vi "HMI_GetPaths.vi"(11 "Main Root Path":path) -> (1 "Default Paths":path[](array[path])=[path "C:/AllenProjects/PWC-OLS/$ReportFiles", path "C:/AllenProjects/PWC-OLS/$ConfigFiles"], 2 "Root Path":path=path "C:/AllenProjects/PWC-OLS", 3 "vi path":path)   [LabVIEW 2024]
doc: "Use to create relative paths to make the program portable.I\n\niNPUTS\nRelative Path is the name of the folder where to begin the file open dialog.\nRoot Name is the String name of the Root folder of this program.\n\nOUTPUS\nFile Path Path to the Opened File\nRoot Path Path to the root Folder\nFile Name String name less Path and extension."
panel:
  in  "Default Relative Paths":path[](array[path])=[path "$ReportFiles", path "$ConfigFiles"]
  in  "Reg Key Srting":string[](array[string])=["Report Files Path", "Config Files Path"]
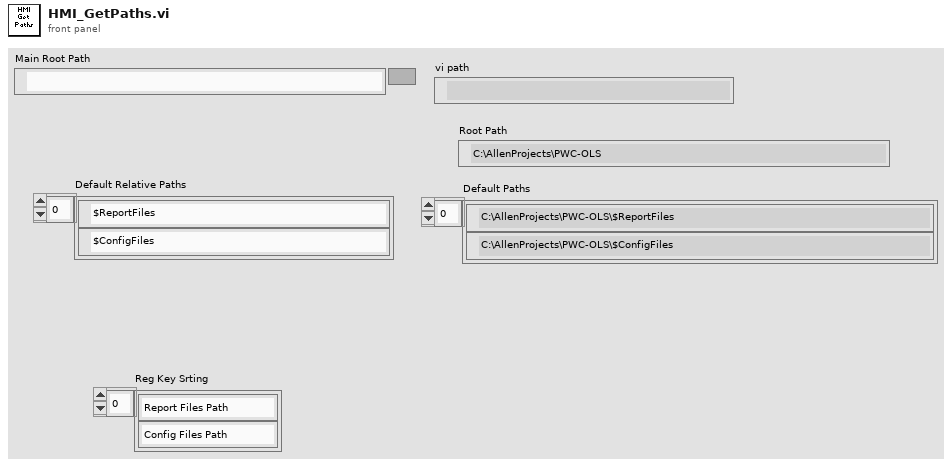
[diagram p1: front panel]
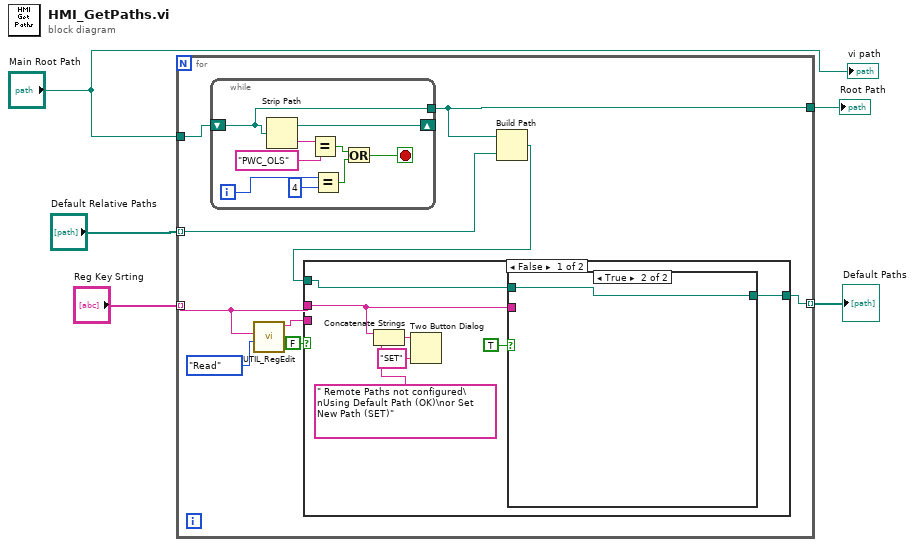
[diagram p0: block diagram]
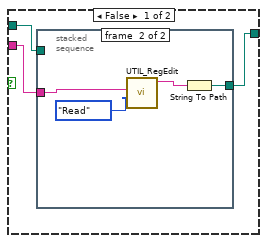
[diagram p2: hidden frame]
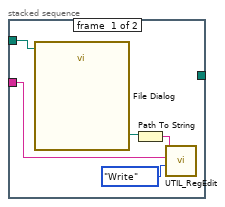
[diagram p3: hidden frame]
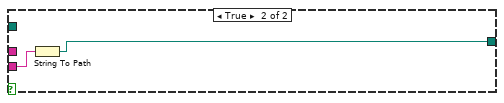
[diagram p4: hidden frame]
diagram:
  n1 = for {
    tunnel: [w6] -> w5
    tunnel: "Default Relative Paths" -> [w14] mode=indexing
    tunnel: [w10] -> w3 mode=indexing
    tunnel: "Reg Key Srting" -> [w9] mode=indexing
    tunnel: "Main Root Path" -> [w7]
    n2 = while {
      shift-right: [w23] -> _
      shift-left: w7 -> [w22]
      tunnel: [w22] -> w6
      i -> [w17]
      stop <- w15 stop-if-true
      n3 = Strip Path(path=w22) -> (stripped path=w23:path, name=w21:string)
      n4 = Equal?(x=w21, y="PWC_OLS") -> (x = y?=w19:bool)
      n5 = Equal?(x=w17, y=4) -> (x = y?=w18:bool)
      n6 = Or(x=w19, y=w18) -> (x .or. y?=w15:bool)
    }
    n7 = call "UTIL_RegEdit.vi"("Mode"=enum16{"Write", "Read", "Delete"}."Read", "String Name"=w9) -> ("Value Read"=w12:string)  [unwired: 8 in, 1 out]
    n8 = Build Path(base path=w6, name or relative path=w14) -> (appended path=w11:path)
    n9 = case shown="False" FALSE {
      tunnel: w12 -> [_ w45]
      tunnel: [w26 w44] -> w10
      tunnel: w11 -> [w27 _]
      tunnel: w9 -> [w25 _]
      frame False {
        n10 = Concatenate Strings(w25, " Remote Paths not configured\nUsing Default Path (OK)\nor Set New Path (SET)") -> (w29:string)
        n11 = Two Button Dialog(message=w29, 1:"SET" ("F button name (\"Cancel\")")) -> ()  [unwired: 1 in, 1 out]
        n12 = case shown="True" TRUE {
          tunnel: [w31 w43] -> w26
          tunnel: w27 -> [w33 w43]
          tunnel: w25 -> [w32 _]
          frame False {
            n13 = stacked-sequence {
              tunnel: w33 -> [w35 _]
              tunnel: w32 -> [w36 w40]
              tunnel: [_ w39] -> w31
              frame #0 {
                n14 = call "File Dialog"("start path"=w35) -> ("selected path"=w34:path)  [unwired: 11 in, 3 out]
                n15 = Path To String(path=w34) -> (string=w37:string)
                n16 = call "UTIL_RegEdit.vi"("Mode"=enum16{"Write", "Read", "Delete"}."Write", "String Name"=w36, "String Value"=w37) -> ()  [unwired: 7 in, 2 out]
              }
              frame #1 {
                n17 = call "UTIL_RegEdit.vi"("Mode"=enum16{"Write", "Read", "Delete"}."Read", "String Name"=w40) -> ("Value Read"=w42:string)  [unwired: 8 in, 1 out]
                n18 = String To Path(string=w42) -> (path=w39:path)
              }
            }
          }
          frame True {
          }
        }
      }
      frame True {
        n19 = String To Path(string=w45) -> (path=w44:path)
      }
    }
  }
  "Root Path" <- w5
  "Default Paths" <- w3
  "vi path" <- "Main Root Path"
